vi "get inverseSurface.vi"(8 "error in":errorcluster, 11 "Material-Scheme in":refnum<class "Material-Scheme.lvclass">) -> (0 "error out":errorcluster, 2 "inverseSurface":u32(colorbox), 3 "Material-Scheme out":refnum<class "Material-Scheme.lvclass">)   [LabVIEW 2021, in "TSC Material Theme.lvlib" / "Material-Scheme.lvclass"]
doc: "get the value for the color from the scheme class: inverseSurface\n\n<b>Code Developed By:</b> +\nDaniel Coons +\nTechnology Service Corporation +\nwww.tsc.com/atcs"
uses:
  Material-Scheme.lvclass
  Material-Scheme.lvclass/Material-Scheme.ctl
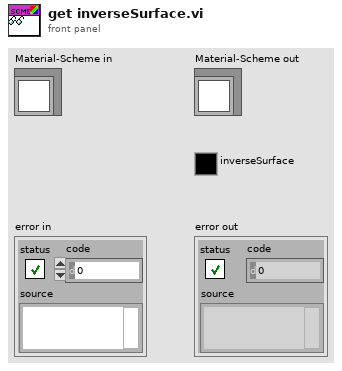
[diagram p1: front panel]
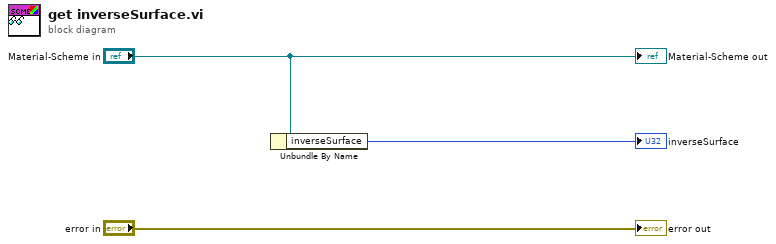
[diagram p0: block diagram]
diagram:
  n1 = Unbundle By Name("Material-Scheme in") -> ("inverseSurface"=→"inverseSurface":u32)
  "error out" <- "error in"
  "Material-Scheme out" <- "Material-Scheme in"
